vi "CD Init_Prepare Async Data.vi"(8 "error in (no error)":errorcluster, 10 "Card Parameters (in)":T1, 11 "Channels In":T19[](array[typedef]) {"RTs"."Mode Codes"."param item refs" format="%.0x"; "RTs"."Mode Codes"."Timestamp Channel Data Reference" format="%.0x"; "RTs"."subAddresses"."param item refs" format="%.0x"; "RTs"."subAddresses"."Timestamp Channel Data Reference" format="%.0x"; "RTs"."Status Channel Data Reference" format="%.0x"; "RTs"."Command Channels Refs" format="%.0x"; "BC"."Acyclic Frames Trigger Channels Refs" format="%.0x"; "BC"."Command Channels Refs" format="%.0x"; "BC"."messages"."Timestamp Channel Data Reference" format="%.0x"; "BC"."messages"."Status Channel Data Refs" format="%.0x"; "BC"."messages"."param item refs" format="%.0x"; "BC"."messages"."param Block Data Refs"."Data Reference" format="%.0x"}) -> (0 "error out":errorcluster, 3 "RT Async Data":T3 {"Map (MC Tx)"."Word Data Reference" format="%.0x"; "Map (MC Rx)"."Channel Data Reference" format="%.0x"; "Map (RT Command Channels)"."RT Command Channel Ref" format="%.0x"; "MAP (BC Acyclic Messages Trigger)"."Acyclic Message Trigger Channel Ref" format="%.0x"; "Map (Bc Command Channels)"."BC Command Channel Ref" format="%.0x"; "Map (RT to ..)"."Word Data Reference" format="%.0x"; "Map (BC to RT)"."Channel Data Reference" format="%.0x"})   [LabVIEW 2020, in "Ballard MIL-1553 Engine.lvlib"]
uses:
  Ballard MIL-1553 Engine.lvlib
  Shared/Controls and Global/RT Channel.ctl
  Shared/Controls and Global/RT BC.ctl
  <vilib>/NI VeriStand/Custom Device API/Custom Device Item Ref.ctl
  Shared/Controls and Global/RT Message.ctl
  Shared/Controls and Global/RT messageType.ctl
  Shared/Controls and Global/RT CWD1.ctl
  Shared/Controls and Global/RT CWD2.ctl
  <vilib>/NI VeriStand/Custom Device API/Data Reference.ctl
  <vilib>/NI VeriStand/Custom Device API/Block Data Reference.ctl
  Shared/EncodeDecode/_typedefs/parameter_config_type.ctl
  Shared/EncodeDecode/_typedefs/parameter_config_type_type.ctl
  Shared/EncodeDecode/_typedefs/parameter_config_encoding_type.ctl
  Shared/Controls and Global/RT Remote Terminal.ctl
  Shared/Controls and Global/RT Remote Terminal_rtMode.ctl
  Shared/Controls and Global/RT Remote Terminal_RT subAddress.ctl
  Shared/Controls and Global/RT Remote Terminal_RT direction.ctl
  Shared/Controls and Global/RT Remote Terminal_RT Mode Code.ctl
  Controls/RT Async Data.ctl
  Controls/RT Async_Map BC2RT.ctl
  Controls/RT Async_Map_Type.ctl
  Controls/RT Async_Raw Values.ctl
  Controls/RT Async_Raw Values to Messages Index_Association.ctl
  Controls/Asynchronous - Parameter map_type.ctl
  Controls/RT Async_Map RT2BC.ctl
  Controls/RT Async_Map RTs Status.ctl
  Controls/RT Async_Map BC Command Channels.ctl
  Controls/RT Async_Map BC Acyclic Messages Trigger.ctl
  Controls/RT Async_Map RT Command Channels.ctl
  Controls/Card Parameters.ctl
  Shared/Controls and Global/Initialization Method.ctl
  <vilib>/NI VeriStand/Custom Device API/Custom Device API.lvlib
  Shared/Ballard 1553 Shared.lvlib
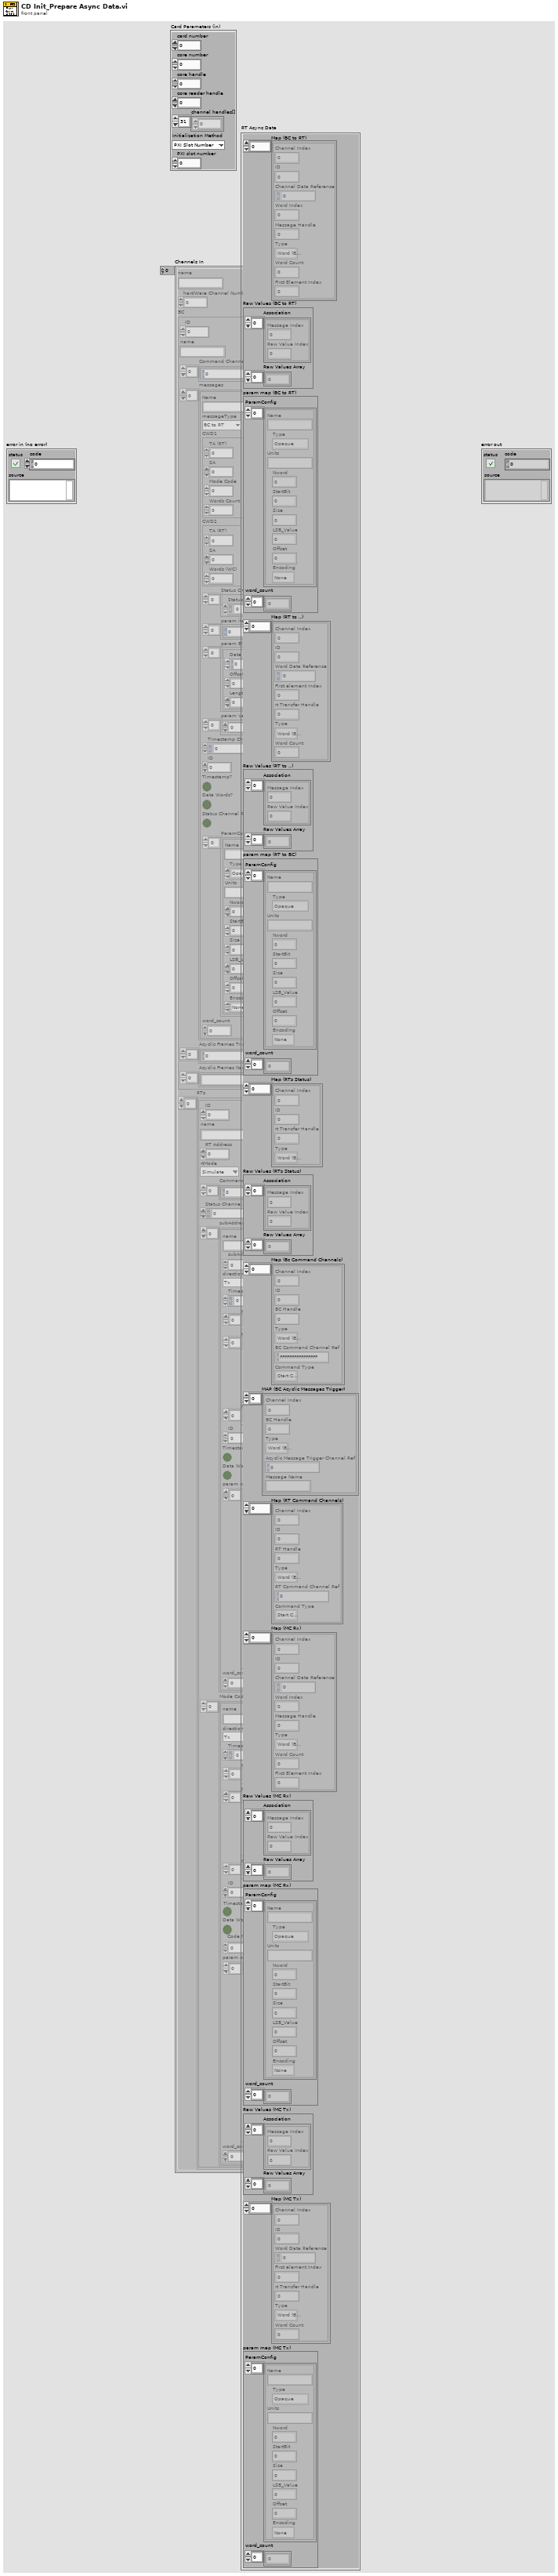
[diagram p1: front panel]
types:
  T1 = typedef "Ballard MIL-1553 Engine.lvlib/Card Parameters.ctl" = cluster{"card number":i32, "core number":i32, "core handle":u64, "core reader handle":u64, "channel handles[]":u64[], "Initialization Method":T2, "PXI slot number":i32}
  T2 = typedef "Ballard 1553 Shared.lvlib/Initialization Method.ctl" = enum16{"PXI Slot Number", "Card Number"}
  T3 = typedef "Ballard MIL-1553 Engine.lvlib/RT Async Data.ctl" = cluster{"Map (BC to RT)":T4[], "Raw Values (BC to RT)":T7, "param map (BC to RT)":T9, "Map (RT to ..)":T13[], "Raw Values (RT to ..)":T7, "param map (RT to BC)":T9, "Map (RTs Status)":T14[], "Raw Values (RTs Status)":T7, "Map (Bc Command Channels)":T15[], "MAP (BC Acyclic Messages Trigger)":T17[], "Map (RT Command Channels)":T18[], "Map (MC Rx)":T4[], "Raw Values (MC Rx)":T7, "param map (MC Rx)":T9, "Raw Values (MC Tx)":T7, "Map (MC Tx)":T13[], "param map (MC Tx)":T9}
  T4 = typedef "Ballard MIL-1553 Engine.lvlib/RT Async_Map BC2RT.ctl" = cluster{"Channel Index":i32, "ID":i32, "Channel Data Reference":T5, "Word Index":i32, "Message Handle":u64, "Type":T6, "Word Count":i32, "First Element Index":i32}
  T5 = typedef "Custom Device API.lvlib/Data Reference.ctl" = i32
  T6 = typedef "Ballard MIL-1553 Engine.lvlib/RT Async_Map_Type.ctl" = enum16{"Word (BC to RT)", "Word (MC (Rx))", "Acyclic Message Trigger", "Word (RT to ..)", "Word (RT to RT)", "Word (MC (Tx))", "RT Status", "BC Commands", "RT Commands"}
  T7 = typedef "Ballard MIL-1553 Engine.lvlib/RT Async_Raw Values.ctl" = cluster{"Association":T8[], "Raw Values Array":u16[]}
  T8 = typedef "Ballard MIL-1553 Engine.lvlib/RT Async_Raw Values to Messages Index_Association.ctl" = cluster{"Message Index":i32, "Raw Value Index":i32}
  T9 = typedef "Ballard MIL-1553 Engine.lvlib/Asynchronous - Parameter map_type.ctl" = cluster{"ParamConfig":T10[], "word_count":u8[]}
  T10 = typedef "parameter_config_type.ctl" = cluster{"Name":string, "Type":T11, "Units":string, "Nword":i32, "StartBit":i32, "Size":i32, "LSB_Value":i32, "Offset":i32, "Encoding":T12}
  T11 = typedef "parameter_config_type_type.ctl" = enum16{"Opaque", "Enum", "Float", "Integer", "Bcd", "Bool"}
  T12 = typedef "parameter_config_encoding_type.ctl" = enum16{"None", "2-complement", "Unsigned"}
  T13 = typedef "Ballard MIL-1553 Engine.lvlib/RT Async_Map RT2BC.ctl" = cluster{"Channel Index":i32, "ID":i32, "Word Data Reference":T5, "First element Index":i32, "rt Transfer Handle":u64, "Type":T6, "Word Count":i32}
  T14 = typedef "Ballard MIL-1553 Engine.lvlib/RT Async_Map RTs Status.ctl" = cluster{"Channel Index":i32, "ID":i32, "rt Transfer Handle":u64, "Type":T6}
  T15 = typedef "Ballard MIL-1553 Engine.lvlib/RT Async_Map BC Command Channels.ctl" = cluster{"Channel Index":i32, "ID":i32, "BC Handle":u64, "Type":T6, "BC Command Channel Ref":T16, "Command Type":enum16{"Start Command", "Stop Command"}}
  T16 = typedef "Custom Device API.lvlib/Custom Device Item Ref.ctl" = u64
  T17 = typedef "Ballard MIL-1553 Engine.lvlib/RT Async_Map BC Acyclic Messages Trigger.ctl" = cluster{"Channel Index":i32, "BC Handle":u64, "Type":T6, "Acyclic Message Trigger Channel Ref":T16, "Message Name":string}
  T18 = typedef "Ballard MIL-1553 Engine.lvlib/RT Async_Map RT Command Channels.ctl" = cluster{"Channel Index":i32, "ID":i32, "RT Handle":u64, "Type":T6, "RT Command Channel Ref":T16, "Command Type":enum16{"Start Command", "Stop Command"}}
  T19 = typedef "Ballard 1553 Shared.lvlib/RT Channel.ctl" = cluster{"name":string, "hardWare Channel Number":u16, "BC":T20, "RTs":T26[]}
  T20 = typedef "Ballard 1553 Shared.lvlib/RT BC.ctl" = cluster{"ID":i32, "name":string, "Command Channels Refs":T16[], "messages":T21[], "Acyclic Frames Trigger Channels Refs":T16[], "Acyclic Frames Names":string[]}
  T21 = typedef "Ballard 1553 Shared.lvlib/RT Message.ctl" = cluster{"Name":string, "messageType":T22, "CWD1":T23, "CWD2":T24, "Status Channel Data Refs":T5[], "param item refs":T16[], "param Block Data Refs":T25[], "param Values Array":u16[], "Timestamp Channel Data Reference":T5, "ID":i32, "Timestamp?":bool, "Data Words?":bool, "Status Channel Ref?":bool, "ParamConfig":T10[], "word_count":u8}
  T22 = typedef "Ballard 1553 Shared.lvlib/RT messageType.ctl" = enum16{"BC to RT", "RT to BC", "RT to RT", "MC (Rx)", "MC (Tx)"}
  T23 = typedef "Ballard 1553 Shared.lvlib/RT CWD1.ctl" = cluster{"TA (RT)":i8, "SA":i8, "Mode Code":i8, "Words Count":i8}
  T24 = typedef "Ballard 1553 Shared.lvlib/RT CWD2.ctl" = cluster{"TA (RT)":i8, "SA":i8, "Words (WC)":i8}
  T25 = typedef "Custom Device API.lvlib/Block Data Reference.ctl" = cluster{"Data Reference":T5, "Offset":u64, "Length":u64}
  T26 = typedef "Ballard 1553 Shared.lvlib/RT Remote Terminal.ctl" = cluster{"ID":i32, "name":string, "RT Address":i32, "rtMode":T27, "Command Channels Refs":T16[], "Status Channel Data Reference":T5, "subAddresses":T28[], "Mode Codes":T30[]}
  T27 = typedef "Ballard 1553 Shared.lvlib/RT Remote Terminal_rtMode.ctl" = enum16{"Simulate", "Monitor", "Disable"}
  T28 = typedef "Ballard 1553 Shared.lvlib/RT Remote Terminal_RT subAddress.ctl" = cluster{"name":string, "subAddress":i8, "direction":T29, "Timestamp Channel Data Reference":T5, "param value array":u16[], "param blocj data refs":T25[], "param item refs":T16[], "ID":i32, "Timestamp?":bool, "Data Words?":bool, "param config":T10[], "word_count":u8}
  T29 = typedef "Ballard 1553 Shared.lvlib/RT Remote Terminal_RT direction.ctl" = enum16{"Tx", "Rx"}
  T30 = typedef "Ballard 1553 Shared.lvlib/RT Remote Terminal_RT Mode Code.ctl" = cluster{"name":string, "direction":T29, "Timestamp Channel Data Reference":T5, "param values array":u16[], "param block data refs":T25[], "param item refs":T16[], "ID":i32, "Timestamp?":bool, "Data Words?":bool, "Code Number":i32, "param config":T10[], "word_count":u8}
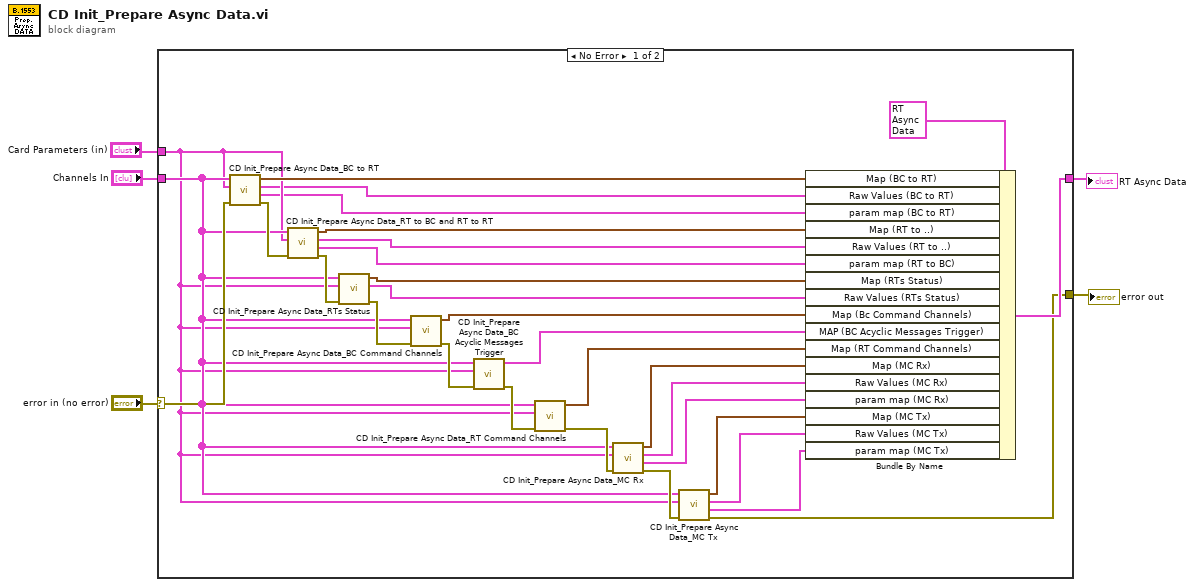
[diagram p0: block diagram]
diagram:
  n1 = case shown="No Error" "error in (no error)" {
    selector: "error in (no error)" -> [w34 w36]
    tunnel: [w15 w36] -> w4
    tunnel: "Channels In" -> [w12 _]
    tunnel: "Card Parameters (in)" -> [w11 _]
    tunnel: [w35 _] -> w1
    frame No Error {
      n2 = call "CD Init_Prepare Async Data_BC to RT.vi"("error in (no error)"=w34, "Card Parameters (in)"=w11, "Channels In"=w12) -> ("error out"=w29:errorcluster, "param map (BC to RT)"=w9:T9, "Raw Values (BC to RT)"=w10:T7, "Map (BC to RT)"=w32:T4[])  [unwired: 5 in]
      n3 = call "CD Init_Prepare Async Data_RT to BC and RT to RT.vi"("error in (no error)"=w29, "Card Parameters (in)"=w11, "Channels In"=w12) -> ("error out"=w28:errorcluster, "param map (RT to BC)"=w8:T9, "Raw Values (RT to BC)"=w30:T7, "Map (RT to BC)"=w31:T13[])  [unwired: 5 in]
      n4 = call "CD Init_Prepare Async Data_RTs Status.vi"("error in (no error)"=w28, "Card Parameters (in)"=w11, "Channels In"=w12) -> ("error out"=w25:errorcluster, "Raw Values (RTs Status)"=w26:T7, "Map (RTs Status)"=w27:T14[])  [unwired: 6 in]
      n5 = call "CD Init_Prepare Async Data_BC Command Channels.vi"("error in (no error)"=w25, "Card Parameters (in)"=w11, "Channels In"=w12) -> ("error out"=w23:errorcluster, "Map (Bc Command Channels)"=w24:T15[])  [unwired: 7 in]
      n6 = call "CD Init_Prepare Async Data_BC Acyclic Messages Trigger.vi"("error in (no error)"=w23, "Card Parameters (in)"=w11, "Channels In"=w12) -> ("error out"=w22:errorcluster, "MAP (BC Acyclic Messages Trigger)"=w21:T17[])  [unwired: 7 in]
      n7 = call "CD Init_Prepare Async Data_RT Command Channels.vi"("error in (no error)"=w22, "Card Parameters (in)"=w11, "Channels In"=w12) -> ("error out"=w19:errorcluster, "Map (RT Command Channels)"=w20:T18[])  [unwired: 7 in]
      n8 = call "CD Init_Prepare Async Data_MC Rx.vi"("error in (no error)"=w19, "Card Parameters (in)"=w11, "Channels In"=w12) -> ("error out"=w16:errorcluster, "param map (MC Rx)"=w7:T9, "Raw Values (MC Rx)"=w17:T7, "Map (MC Rx)"=w18:T4[])  [unwired: 5 in]
      n9 = call "CD Init_Prepare Async Data_MC Tx.vi"("error in (no error)"=w16, "Card Parameters (in)"=w11, "Channels In"=w12) -> ("error out"=w15:errorcluster, "param map (MC Rx)"=w6:T9, "Raw Values (RT to BC)"=w13:T7, "Map (MC Tx)"=w14:T13[])  [unwired: 5 in]
      n10 = Bundle By Name(cluster=T3 {"Map (BC to RT)"=[], "Raw Values (BC to RT)"={"Association"=[], "Raw Values Array"=[]}, "param map (BC to RT)"={"ParamConfig"=[], "word_count"=[]}, "Map (RT to ..)"=[], "Raw Values (RT to ..)"={"Association"=[], "Raw Values Array"=[]}, "param map (RT to BC)"={"ParamConfig"=[], "word_count"=[]}, "Map (RTs Status)"=[], "Raw Values (RTs Status)"={"Association"=[], "Raw Values Array"=[]}, "Map (Bc Command Channels)"=[], "MAP (BC Acyclic Messages Trigger)"=[], "Map (RT Command Channels)"=[], "Map (MC Rx)"=[], "Raw Values (MC Rx)"={"Association"=[], "Raw Values Array"=[]}, "param map (MC Rx)"={"ParamConfig"=[], "word_count"=[]}, "Raw Values (MC Tx)"={"Association"=[], "Raw Values Array"=[]}, "Map (MC Tx)"=[], "param map (MC Tx)"={"ParamConfig"=[], "word_count"=[]}} ("RT Async Data"), "Map (BC to RT)"=w32, "Raw Values (BC to RT)"=w10, "param map (BC to RT)"=w9, "Map (RT to ..)"=w31, "Raw Values (RT to ..)"=w30, "param map (RT to BC)"=w8, "Map (RTs Status)"=w27, "Raw Values (RTs Status)"=w26, "Map (Bc Command Channels)"=w24, "MAP (BC Acyclic Messages Trigger)"=w21, "Map (RT Command Channels)"=w20, "Map (MC Rx)"=w18, "Raw Values (MC Rx)"=w17, "param map (MC Rx)"=w7, "Map (MC Tx)"=w14, "Raw Values (MC Tx)"=w13, "param map (MC Tx)"=w6) -> (w35:T3)
    }
    frame Error {
    }
  }
  "error out" <- w4
  "RT Async Data" <- w1
